vi "Vision Processing.vi"(4 "error in (no error)":errorcluster, 7 "Image Size":T1=enum."320x240") -> ()   [LabVIEW 2013]
doc: "This VI runs in parallel to other tasks. It gets images from the camera, processes them for color or shape and use that information to affect robot behavior."
uses:
  <vilib>/Rock Robotics/WPI/Camera/WPI_CameraImageSize.ctl
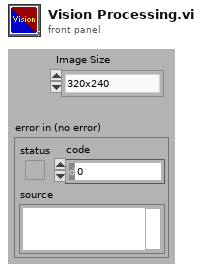
[diagram p1: front panel]
types:
  T1 = typedef "WPI_CameraImageSize.ctl" = enum16{"640x480", "320x240", "160x120"}
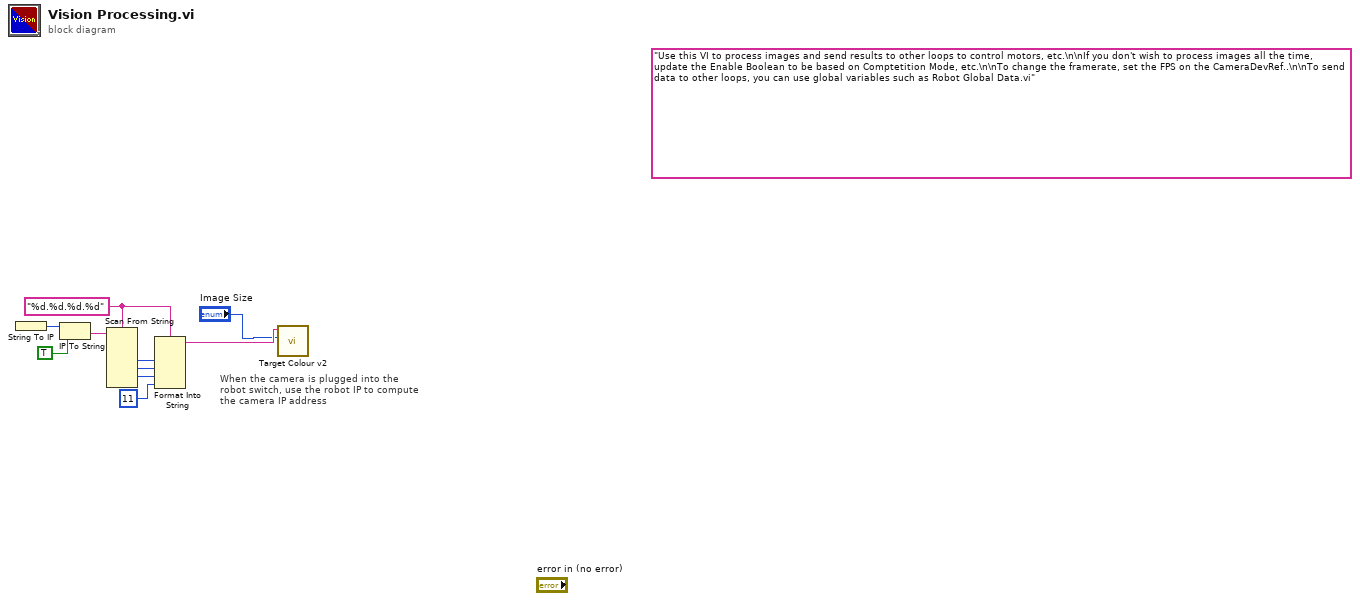
[diagram p0: block diagram]
diagram:
  w3 = "%d.%d.%d.%d" ("format string")
  (unwired) "Use this VI to process images and send results to other loops to control motors, etc.\n\nIf you don't wish to process images all the time, update the Enable Boolean to be based on Comptetition Mode, etc.\n\nTo change the framerate, set the FPS on the CameraDevRef..\n\nTo send data to other loops, you can use global variables such as Robot Global Data.vi"
  # "When the camera is plugged into the\nrobot switch, use the robot IP to compute\nthe camera IP address"
  n1 = String To IP() -> (0:w10:u32)  [unwired: 1 in]
  n2 = IP To String(1:TRUE ("dot notation? (F)"), 2:w10) -> (0:w8:string)
  n3 = Scan From String(format string=w3, input string=w8) -> (output 1=w7:i32, output 2=w6:i32, output 3=w5:i32)  [unwired: 7 in, 3 out]
  n4 = Format Into String(format string=w3, w7, w6, w5, 11 ("Compression")) -> (resulting string=w2:string)  [unwired: 2 in, 1 out]
  n5 = call "Target Colour v2.vi"("Camera IP"=w2, "Image Size"="Image Size") -> ()  [unwired: 9 in]
